vi "Create from SQL Record.vi"(8 "error in (no error)":errorcluster, 11 "MySQL Record":variant[](array[variant])) -> (0 "error out":errorcluster, 3 "Banking Record":refnum<class "Banking Record.lvclass">)   [LabVIEW 2018, in "Banking Record.lvclass"]
uses:
  Banking Record.lvclass
  Banking Record.lvclass/Banking Record.ctl
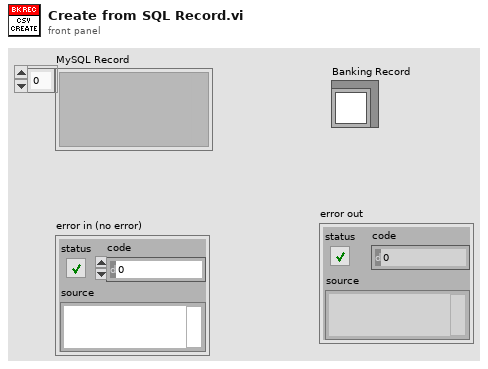
[diagram p1: front panel]
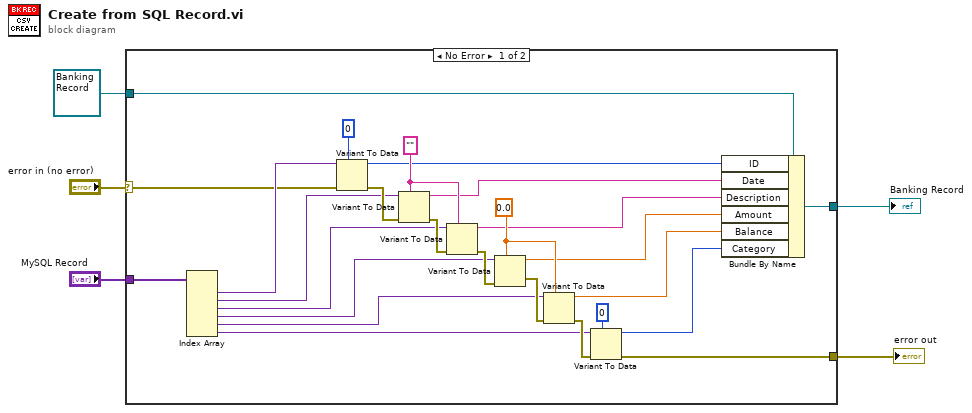
[diagram p0: block diagram]
diagram:
  n1 = case shown="No Error" "error in (no error)" {
    selector: "error in (no error)" -> [w10 w33]
    tunnel: [w31 w32] -> w5
    tunnel: [w8 w33] -> w3
    tunnel: refnum<class "Banking Record.lvclass"> refnum ("Banking Record.lvclass") -> [w20 w32]
    tunnel: "MySQL Record" -> [w9 _]
    frame No Error {
      w18 = 0.0 ("Amount")
      w17 = "" ("type")
      n2 = Index Array(array=w9) -> (element #1=w25:variant, element #2=w7:variant, element #3=w24:variant, element #4=w23:variant, element #5=w22:variant, element #6=w21:variant)  [unwired: 6 in]
      n3 = Variant To Data(error in=w10, type=0 ("id"), Variant=w25) -> (data=w15:i32, error out=w30:errorcluster)
      n4 = Variant To Data(error in=w30, type=w17, Variant=w7) -> (data=w6:string, error out=w26:errorcluster)
      n5 = Variant To Data(error in=w26, type=w17, Variant=w24) -> (data=w16:string, error out=w27:errorcluster)
      n6 = Variant To Data(error in=w27, type=w18, Variant=w23) -> (data=w14:dbl, error out=w28:errorcluster)
      n7 = Variant To Data(error in=w28, type=w18, Variant=w22) -> (data=w13:dbl, error out=w29:errorcluster)
      n8 = Variant To Data(error in=w29, type=0 ("id"), Variant=w21) -> (data=w11:i32, error out=w8:errorcluster)
      n9 = Bundle By Name(cluster=w20, "ID"=w15, "Date"=w6, "Description"=w16, "Amount"=w14, "Balance"=w13, "Category"=w11) -> (w31:refnum<class "Banking Record.lvclass">)
    }
    frame Error {
    }
  }
  "Banking Record" <- w5
  "error out" <- w3
